vi "Read Map.vi"(8 "error in (no error)":errorcluster, 11 "TrafficMap in":refnum<class "TrafficMap.lvclass">) -> (0 "error out":errorcluster, 2 "Map":u16[][](array[numeric]), 3 "TrafficMap out":refnum<class "TrafficMap.lvclass">)   [LabVIEW 2017, in "TrafficMap.lvclass"]
uses:
  TrafficMap.lvclass
  TrafficMap.lvclass/TrafficMap.ctl
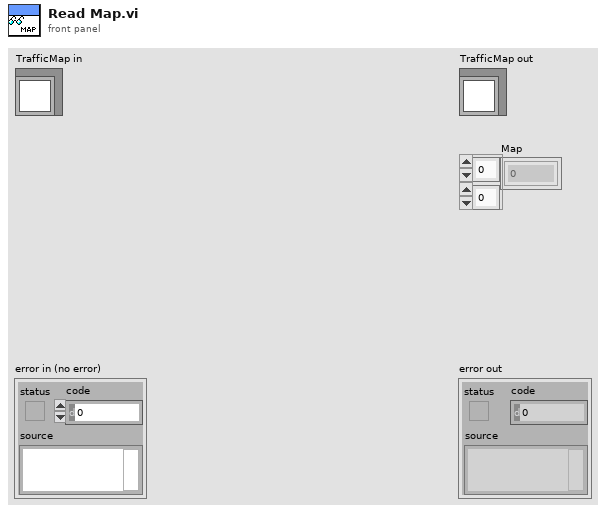
[diagram p1: front panel]
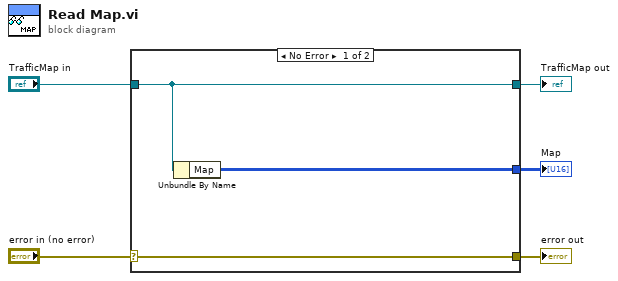
[diagram p0: block diagram]
diagram:
  n1 = case shown="No Error" "error in (no error)" {
    selector: "error in (no error)" -> [w8 w9]
    tunnel: [w8 w9] -> w4
    tunnel: [w7 w10] -> w2
    tunnel: "TrafficMap in" -> [w7 w10]
    tunnel: [w6 _] -> w1
    frame No Error {
      n2 = Unbundle By Name(w7) -> ("Map"=w6:u16[][])
    }
    frame Error {
    }
  }
  "error out" <- w4
  "TrafficMap out" <- w2
  "Map" <- w1
